vi "sv_Compute Swept Sine Harmonic Distortion.vi"(4 "harmonic mapping":u32[](array[numeric]), 5 "unscaled \nresponse magnitude":dbl format="%.2f", 6 "maximum THD harmonic":u32, 7 "reset":bool, 8 "unscaled measurements in":T1 {"harmonic components [ratio]" format="%.2f"; "THD [ratio]" format="%.2f"; "FRF Measurements"."Im [response]" format="%.2f"; "FRF Measurements"."Re [response]" format="%.2f"; "FRF Measurements"."Im [stimulus]" format="%.2f"; "FRF Measurements"."Re [stimulus]" format="%.2f"; "RMS response" format="%.2f"; "RMS stimulus" format="%.2f"}, 10 "frequency (normalized)":dbl format="%.2f", 11 "windowed data":cluster{"stimulus":dbl[], "response":dbl[]} {"response" format="%.2f"; "stimulus" format="%.2f"}) -> (0 "unscaled measurements out":T1 {"harmonic components [ratio]" format="%.2f"; "THD [ratio]" format="%.2f"; "FRF Measurements"."Im [response]" format="%.2f"; "FRF Measurements"."Re [response]" format="%.2f"; "FRF Measurements"."Im [stimulus]" format="%.2f"; "FRF Measurements"."Re [stimulus]" format="%.2f"; "RMS response" format="%.2f"; "RMS stimulus" format="%.2f"}, 3 "dup windowed data":cluster{"stimulus":dbl[], "response":dbl[]} {"response" format="%.2f"; "stimulus" format="%.2f"})   [LabVIEW 2017, in "SoundVib_SweptSine.lvlib"]
uses:
  <vilib>/addons/Sound and Vibration/svt_Swept Sine/SoundVib_SweptSine.lvlib
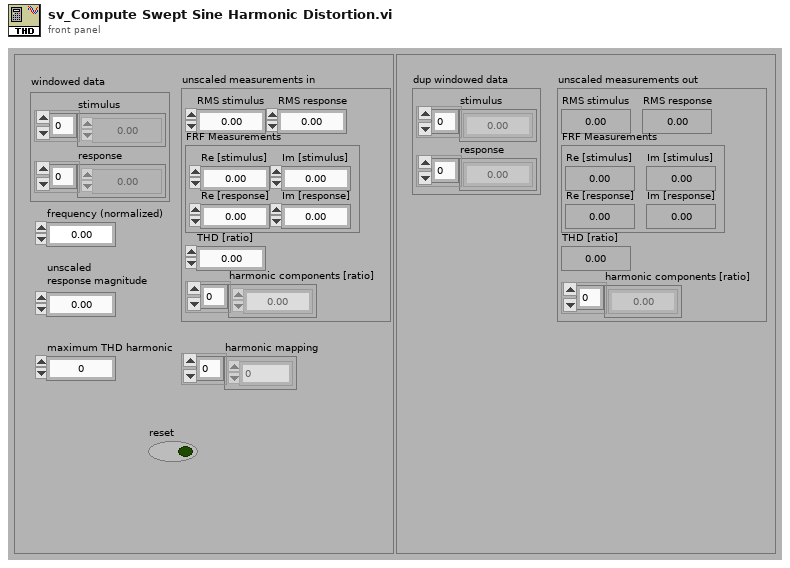
[diagram p1: front panel]
types:
  T1 = cluster{"RMS stimulus":dbl, "RMS response":dbl, "FRF Measurements":cluster{"Re [stimulus]":dbl, "Im [stimulus]":dbl, "Re [response]":dbl, "Im [response]":dbl}, "THD [ratio]":dbl, "harmonic components [ratio]":dbl[]}
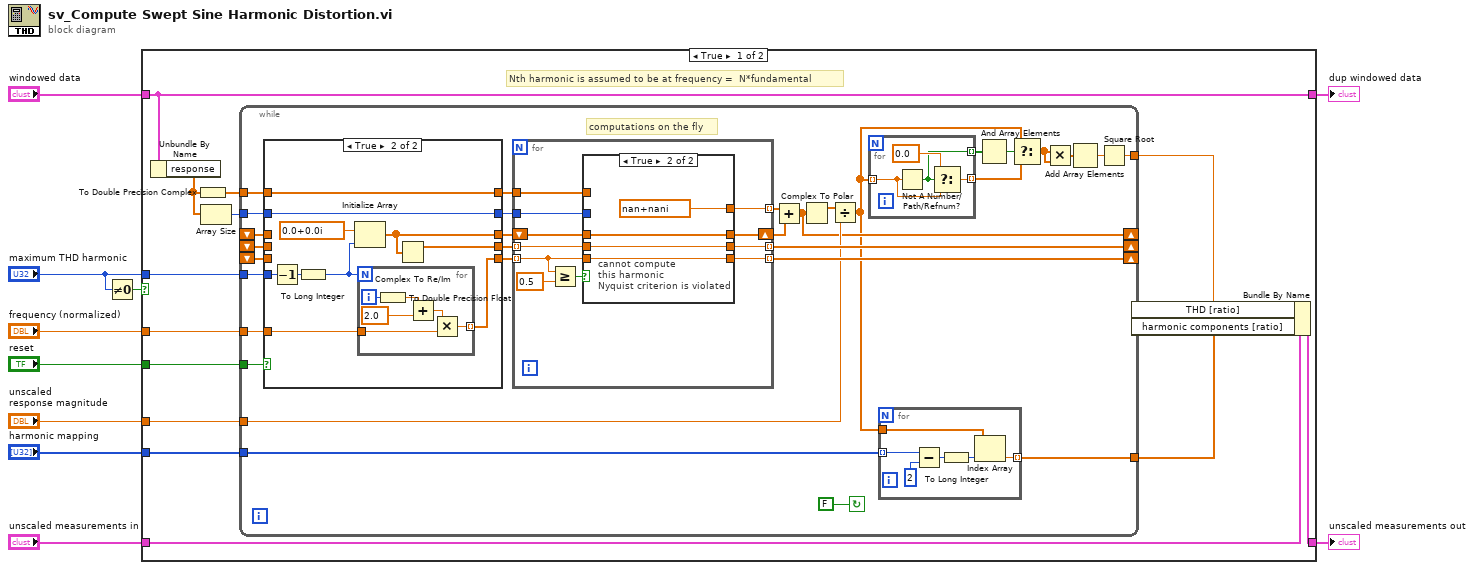
[diagram p0: block diagram]
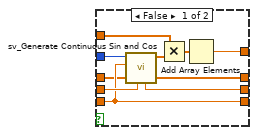
[diagram p3: hidden frame]
diagram:
  n1 = Not Equal To 0?(x="maximum THD harmonic") -> (x != 0?=w4:bool)
  n2 = case shown="True" w4 {
    tunnel: "reset" -> [w23 _]
    tunnel: "windowed data" -> [w15 w111]
    tunnel: "unscaled \nresponse magnitude" -> [w22 _]
    tunnel: [w15 w111] -> w8
    tunnel: "unscaled measurements in" -> [w18 w110]
    tunnel: [w17 w110] -> w3
    tunnel: "harmonic mapping" -> [w21 _]
    tunnel: "frequency (normalized)" -> [w20 _]
    tunnel: "maximum THD harmonic" -> [w12 _]
    frame True {
      # "Nth harmonic is assumed to be at frequency =  N*fundamental"
      n3 = Unbundle By Name(w15) -> ("response"=w14:dbl[])
      n4 = To Double Precision Complex(1:w14) -> (0:w16:cdb[])
      n5 = Array Size(array=w14) -> (size(s)=w13:i32)
      n6 = while {
        tunnel: w23 -> [w48]
        tunnel: [w52] -> w19
        shift-right: [w50] -> _
        shift-left: _ -> [w51]
        shift-right: [w29] -> _
        shift-left: _ -> [w45]
        tunnel: w21 -> [w33]
        tunnel: w20 -> [w40]
        tunnel: w22 -> [w34]
        tunnel: w13 -> [w42]
        tunnel: w16 -> [w44]
        tunnel: w12 -> [w47]
        shift-right: [w37] -> _
        shift-left: _ -> [w39]
        tunnel: [w30] -> w11
        stop <- FALSE continue-if-true
        # "computations on the fly"
        n7 = case shown="True" w48 {
          tunnel: w47 -> [_ w72]
          tunnel: [w63 w70] -> w46
          tunnel: [w62 w71] -> w36
          tunnel: w51 -> [w63 _]
          tunnel: w45 -> [w62 _]
          tunnel: w44 -> [w61 w69]
          tunnel: [w61 w69] -> w43
          tunnel: w42 -> [w60 w68]
          tunnel: [w60 w68] -> w41
          tunnel: w40 -> [_ w65]
          tunnel: [w59 w64] -> w38
          tunnel: w39 -> [w59 _]
          frame False {
          }
          frame True {
            n8 = Decrement(x=w72) -> (x-1=w67:u32)
            n9 = To Long Integer(number=w67) -> (32bit integer=w66:i32)
            n10 = Initialize Array(cdb 0.0+0.0i, w66) -> (w71:cdb[])
            n11 = for {
              N: w66 -> [_]
              tunnel: w65 -> [w74]
              tunnel: [w79] -> w64 mode=indexing
              i -> [w78]
              n12 = To Double Precision Float(number=w78) -> (double precision float=w77:dbl)
              n13 = Add(x=w77, y=2.0 ("x")) -> (x+y=w75:dbl)
              n14 = Multiply(x=w75, y=w74) -> (x*y=w79:dbl)
            }
            n15 = Complex To Re/Im(x + iy=w71) -> (x=w70:dbl[])  [unwired: 1 out]
          }
        }
        n16 = for {
          tunnel: w41 -> [w90]
          tunnel: w46 -> [w89] mode=indexing
          tunnel: [w88] -> w50 mode=indexing
          tunnel: w43 -> [w87]
          tunnel: [w86] -> w49 mode=indexing
          tunnel: w38 -> [w83] mode=indexing
          tunnel: [w82] -> w37 mode=indexing
          shift-right: [w80] -> w35
          shift-left: w36 -> [w81]
          n17 = Greater Or Equal?(x=w83, y=0.5) -> (x >= y?=w84:bool)
          n18 = case shown="True" w84 {
            tunnel: w90 -> [w99 _]
            tunnel: w89 -> [w98 w102]
            tunnel: [w97 w102] -> w88
            tunnel: w87 -> [w96 _]
            tunnel: [w95 cdb nan+nani] -> w86
            tunnel: w83 -> [w92 w103]
            tunnel: [w92 w103] -> w82
            tunnel: w81 -> [w91 w100]
            tunnel: [w91 w100] -> w80
            frame False {
              n19 = call <vilib>:"sv_Generate Continuous Sin and Cos.vi"("sin phase in [degrees]"=w98, "frequency [cycles/sample]"=w92, "number of samples"=w99) -> ("cos (theta) + i sin(theta)"=w93:cdb[], "sin phase out [degrees]"=w97:dbl)  [unwired: 7 in]
              n20 = Multiply(x=w96, y=w93) -> (x*y=w94:cdb[])
              n21 = Add Array Elements(numeric array=w94) -> (sum=w95:cdb)
            }
            frame True {
              # "cannot compute\nthis harmonic\nNyquist criterion is violated"
            }
          }
        }
        n22 = Add(x=w49, y=w35) -> (x+y=w29:cdb[])
        n23 = Complex To Polar(r * e^(i*theta)=w29) -> (r=w54:dbl[])  [unwired: 1 out]
        n24 = Divide(x=w54, y=w34) -> (x/y=w26:dbl[])
        n25 = for {
          tunnel: [w56] -> w25 mode=indexing
          tunnel: w26 -> [w57] mode=indexing
          tunnel: [w55] -> w28 mode=indexing
          n26 = Not A Number/Path/Refnum?(number/path/refnum=w57) -> (NaN/Path/Refnum?=w55:bool)
          n27 = Select(t=0.0, s=w55, f=w57) -> (s? t:f=w56:dbl)
        }
        n28 = for {
          tunnel: w26 -> [w109]
          tunnel: [w107] -> w52 mode=indexing
          tunnel: w33 -> [w106] mode=indexing
          n29 = Subtract(x=w106, y=u32 2) -> (x-y=w105:u32)
          n30 = To Long Integer(number=w105) -> (32bit integer=w104:i32)
          n31 = Index Array(array=w109, index=w104) -> (element=w107:dbl)
        }
        n32 = And Array Elements(Boolean array=w28) -> (logical AND=w27:bool)
        n33 = Select(t=w26, s=w27, f=w25) -> (s? t:f=w24:dbl[])
        n34 = Multiply(x=w24, y=w24) -> (x*y=w32:dbl[])
        n35 = Add Array Elements(numeric array=w32) -> (sum=w31:dbl)
        n36 = Square Root(x=w31) -> (sqrt(x)=w30:dbl)
      }
      n37 = Bundle By Name(cluster=w18, "THD [ratio]"=w11, "harmonic components [ratio]"=w19) -> (w17:T1)
    }
    frame False {
    }
  }
  "dup windowed data" <- w8
  "unscaled measurements out" <- w3
